vi "Simple 48-bit Subtracter using DSP48E.vi"(8 "Input Valid":bool=TRUE, 10 "A2":fxp<+/-,48,48>, 11 "A1":fxp<+/-,48,48>) -> (0 "Output Valid":bool=TRUE, 3 "A1-A2":fxp<+/-,48,48>)   [LabVIEW 2012]
doc: "This VI aubtracts two 48-bit numbers using DSP48E. The output is a 48-bit number.\n\nNo overflow logic is coded into the algorithm.\n\n<b> Latency = 4 Ticks </b>\n<b> Resource Usage = 1 DSP48E </b>"
uses:
  <vilib>/rvi/FXPMathLib/basic elements/DSP48E/simVIs/niFpgaDsp48eSimulationState.ctl
  <vilib>/rvi/FXPMathLib/basic elements/DSP48E/subVIs/niFpgaDsp48eType.ctl
  <vilib>/rvi/FXPMathLib/basic elements/DSP48E/subVIs/niFpgaDsp48eAlumodeOpmodeCarryinselState.ctl
  <vilib>/rvi/FXPMathLib/basic elements/DSP48E/subVIs/niFpgaDsp48eUseMultiplierState.ctl
  <vilib>/rvi/FXPMathLib/basic elements/DSP48E/subVIs/niFpgaDsp48eLogicUnitModeState.ctl
  <vilib>/rvi/FXPMathLib/basic elements/DSP48E/subVIs/niFpgaDsp48eSelectPatternState.ctl
  <vilib>/rvi/FXPMathLib/basic elements/DSP48E/subVIs/niFpgaDsp48eSelectMaskState.ctl
  <vilib>/rvi/FXPMathLib/basic elements/DSP48E/subVIs/niFpgaDsp48eAutoresetState.ctl
  <vilib>/rvi/FXPMathLib/basic elements/DSP48E/simVIs/niFpgaDsp48eResets.ctl
  <vilib>/rvi/FXPMathLib/basic elements/DSP48E/simVIs/niFpgaDsp48eEnables.ctl
  <vilib>/rvi/FXPMathLib/basic elements/DSP48E/simVIs/niFpgaDsp48eRegisters.ctl
  <vilib>/rvi/FXPMathLib/basic elements/DSP48E/simVIs/niFpgaDsp48eSimMultiplier.vi
  <vilib>/rvi/FXPMathLib/basic elements/DSP48E/simVIs/niFpgaDsp48eSimArithmetic.vi
  <vilib>/rvi/FXPMathLib/basic elements/DSP48E/simVIs/niFpgaDsp48eSimPatternDetect.vi
  <vilib>/rvi/FXPMathLib/basic elements/DSP48E/simVIs/niFpgaDsp48eSimP.vi
  <vilib>/rvi/FXPMathLib/basic elements/DSP48E/simVIs/niFpgaDsp48eSimUpdateState.vi
  <vilib>/rvi/FXPMathLib/basic elements/DSP48E/simVIs/niFpgaDsp48eCheckMode.vi
  <vilib>/rvi/FXPMathLib/basic elements/DSP48E/simVIs/niFpgaDsp48eReportInvalidMode.vi
  <vilib>/rvi/FXPMathLib/basic elements/FxpDiscreteDelay/XNode/nifxpmath_DiscreteDelay.xnode
  <vilib>/rvi/FXPMathLib/basic elements/DSP48E/XNode/niFpgaDsp48e.xnode
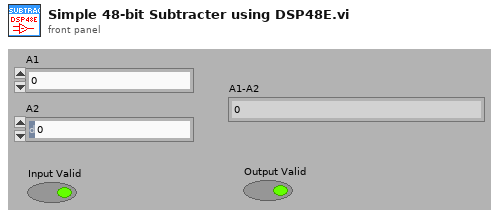
[diagram p1: front panel]
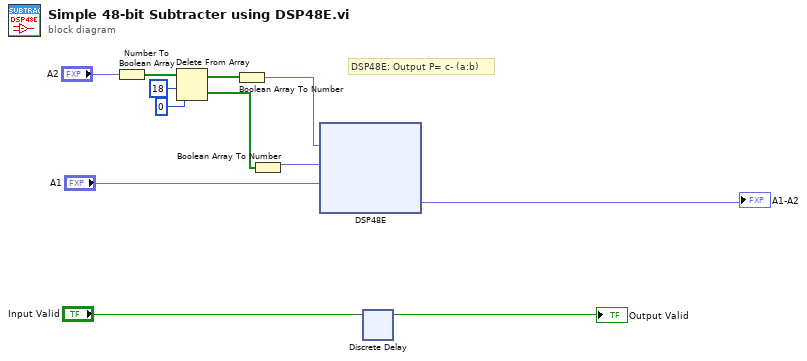
[diagram p0: block diagram]
diagram:
  # "DSP48E: Output P= c- (a:b)"
  n1 = Number To Boolean Array(number="A2") -> (Boolean array=w7:bool[])
  n2 = Delete From Array(array=w7, length=18, index=0) -> (deleted portion=w5:bool[], array with subset deleted=w6:bool[])
  n3 = Boolean Array To Number(Boolean array=w6) -> (number=w8:fxp<+/-,30,30>)
  n4 = Boolean Array To Number(Boolean array=w5) -> (number=w9:fxp<+/-,18,18>)
  n5 = xnode "DSP48E"("a"=w8, "b"=w9, "c"="A1") -> ("p"=→"A1-A2":fxp<+/-,48,48>)
  n6 = xnode "Discrete Delay"("D"="Input Valid") -> ("Q"=→"Output Valid":bool)
